vi "test Check for Invalid Section IDs.vi"(8 "error in (no error)":errorcluster, 11 "TestCase in":refnum<class "Routing and Faulting Scripting Unit Tests.lvclass">) -> (0 "error out":errorcluster, 3 "TestCase out":refnum<class "Routing and Faulting Scripting Unit Tests.lvclass">)   [LabVIEW 2017, in "Routing and Faulting Scripting Unit Tests.lvclass"]
uses:
  Routing and Faulting Scripting Unit Tests.lvclass
  <vilib>/NI Veristand/Custom Device API/Custom Device Item Ref.ctl
  Routing and Faulting Scripting Unit Tests.lvclass/Routing and Faulting Scripting Unit Tests.ctl
  Shared/Alias Mapping.ctl
  <vilib>/addons/_JKI Toolkits/VI Tester/TestCase.llb/TestCase.lvclass
  Routing and Faulting Scripting.lvlib
  Shared/Routing and Faulting Shared.lvlib
  <vilib>/NI VeriStand/Custom Device API/Custom Device API.lvlib
  C:/Program Files (x86)/National Instruments/LabVIEW 2017/vi.lib/addons/_JKI Toolkits/VI Tester/TestCase.llb/TestCase.lvclass
panel:
  in  "Save?":bool
  out "Output Filename":string
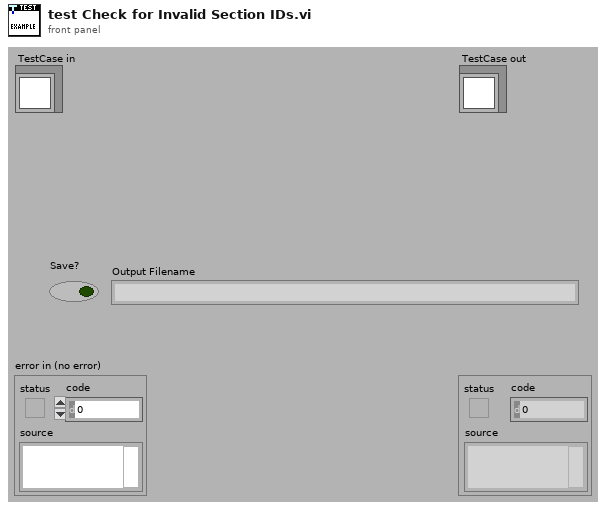
[diagram p1: front panel]
types:
  T1 = typedef "Custom Device API.lvlib/Custom Device Item Ref.ctl" = u64
  T2 = typedef "Routing and Faulting Shared.lvlib/Alias Mapping.ctl" = cluster{"Endpoint":string, "Alias":string}
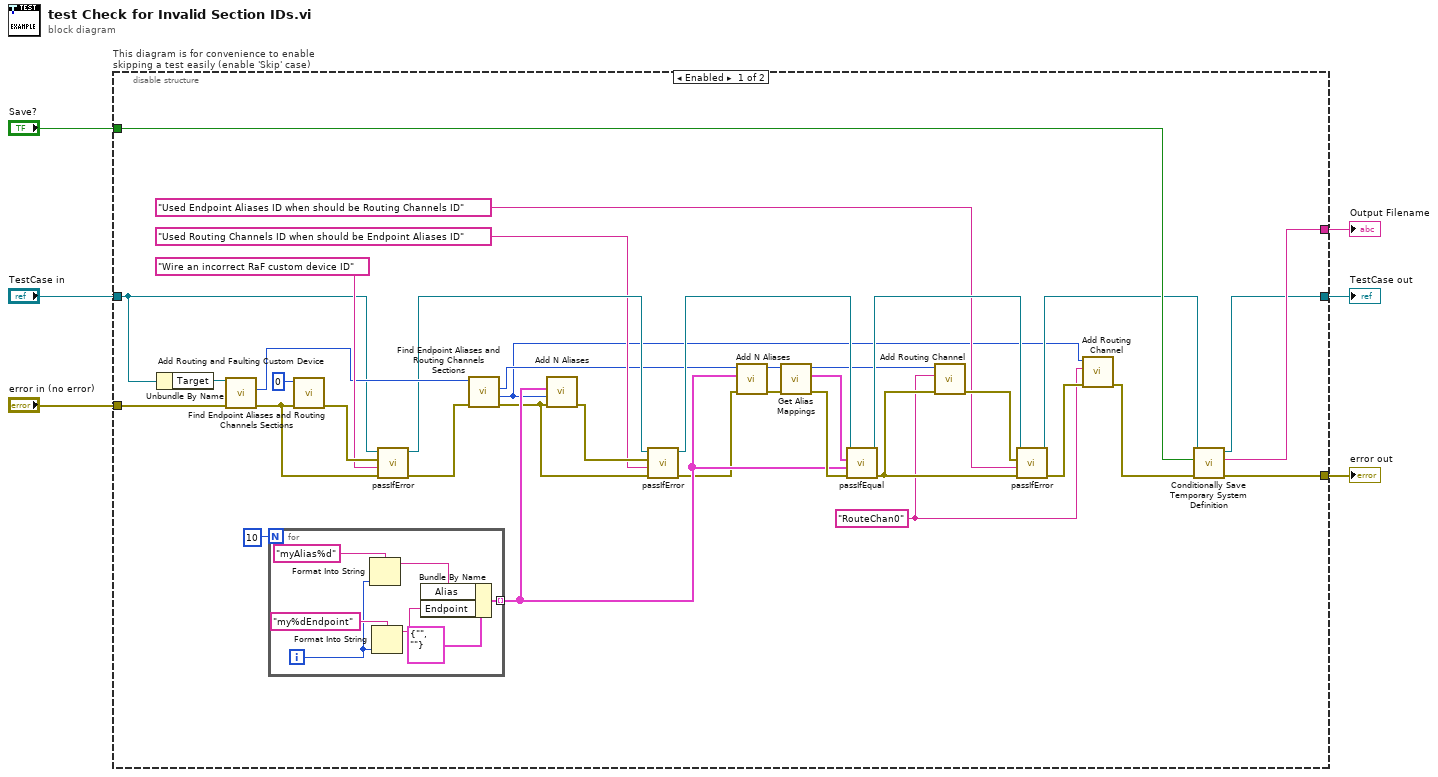
[diagram p0: block diagram]
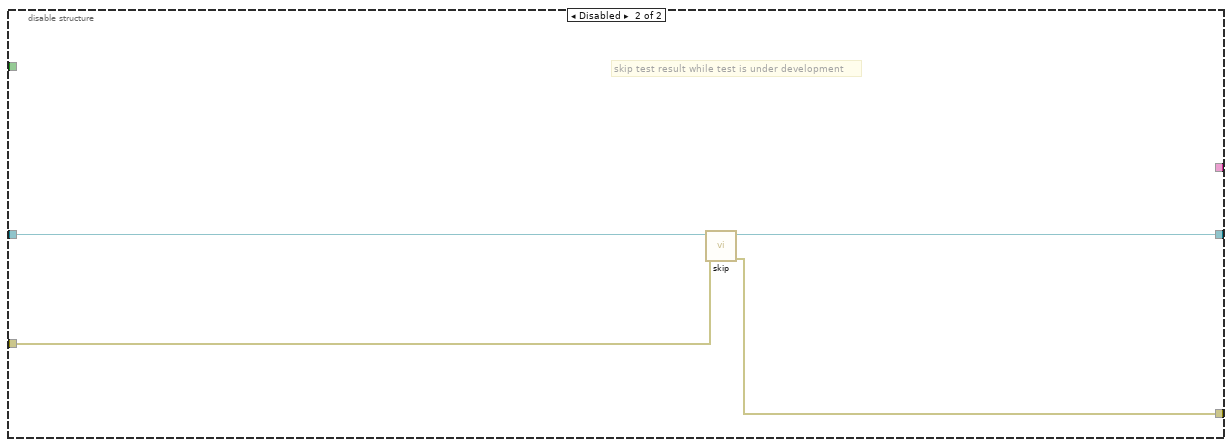
[diagram p2: hidden frame]
diagram:
  n1 = disable-structure "This diagram is for convenience to enable skipping a test easily (enable 'Skip' case)" shown="Enabled" {
    disable-tunnel: "TestCase in" -> [w25 w53]
    disable-tunnel: [w40 w51] -> w3
    disable-tunnel: [w41 w52] -> w5
    disable-tunnel: "error in (no error)" -> [w38 w50]
    disable-tunnel: [w42 _] -> w2
    disable-tunnel: "Save?" -> [w37 _]
    frame Enabled {
      w8 = "RouteChan0" ("Channel Name")
      n2 = Unbundle By Name(w25) -> ("Target"=w39:refnum<k24>)
      n3 = call "Add Routing and Faulting Custom Device.vi"("error in (no error)"=w38, "Target in"=w39) -> ("error out"=w31:errorcluster, "Routing and Faulting Custom Device Ref"=w28:T1)  [unwired: 7 in, 1 out]
      n4 = for {
        N: 10 -> [_]
        tunnel: [w43] -> w24 mode=indexing
        i -> [w47]
        n5 = Format Into String(format string="myAlias%d" ("Alias"), w47) -> (resulting string=w45:string)  [unwired: 2 in, 1 out]
        n6 = Format Into String(format string="my%dEndpoint" ("Alias"), w47) -> (resulting string=w44:string)  [unwired: 2 in, 1 out]
        n7 = Bundle By Name(cluster=T2 {"Endpoint"="", "Alias"=""} ("Alias Mapping"), "Alias"=w45, "Endpoint"=w44) -> (w43:T2)
      }
      n8 = call "Find Endpoint Aliases and Routing Channels Sections.vi"("error in (no error)"=w31, "Routing and Faulting Custom Device Ref in"=T1 0) -> ("error out"=w30:errorcluster)  [unwired: 6 in, 3 out]
      n9 = call-dynamic "passIfError.vi"("error in (no error)"=w31, "task (\"\")"="Wire an incorrect RaF custom device ID" ("task (\"\")"), "error"=w30, "TestCase in"=w25) -> ("error out"=w27:errorcluster, "TestCase out"=w23:refnum<class "Routing and Faulting Scripting Unit Tests.lvclass">)  [unwired: 6 in]
      n10 = call "Find Endpoint Aliases and Routing Channels Sections.vi"("error in (no error)"=w27, "Routing and Faulting Custom Device Ref in"=w28) -> ("error out"=w21:errorcluster, "Routing Channels Ref"=w7:T1, "Endpoint Aliases Ref"=w17:T1)  [unwired: 6 in, 1 out]
      n11 = call "Add N Aliases.vi"("error in (no error)"=w21, "Alias Mappings"=w24, "Endpoint Aliases Ref in"=w7) -> ("error out"=w20:errorcluster)  [unwired: 7 in, 1 out]
      n12 = call-dynamic "passIfError.vi"("error in (no error)"=w21, "task (\"\")"="Used Routing Channels ID when should be Endpoint Aliases ID" ("task (\"\")"), "error"=w20, "TestCase in"=w23) -> ("error out"=w18:errorcluster, "TestCase out"=w22:refnum<class "Routing and Faulting Scripting Unit Tests.lvclass">)  [unwired: 6 in]
      n13 = call "Add N Aliases.vi"("error in (no error)"=w18, "Alias Mappings"=w24, "Endpoint Aliases Ref in"=w17) -> ("error out"=w36:errorcluster, "Endpoint Aliases Ref out"=w35:T1)  [unwired: 7 in]
      n14 = call "Get Alias Mappings.vi"("error in (no error)"=w36, "Endpoint Aliases Ref in"=w35) -> ("error out"=w34:errorcluster, "Alias Mappings"=w33:T2[], "Endpoint Aliases Ref out"=w12:T1)  [unwired: 7 in]
      n15 = call-dynamic "passIfEqual.vi"("error in (no error)"=w34, "y"=w24, "x"=w33, "TestCase in"=w22) -> ("error out"=w14:errorcluster, "TestCase out"=w16:refnum<class "Routing and Faulting Scripting Unit Tests.lvclass">)  [unwired: 6 in]
      n16 = call "Add Routing Channel.vi"("error in (no error)"=w14, "Channel Name"=w8, "Routing Channels Ref in"=w12) -> ("error out"=w13:errorcluster)  [unwired: 6 in, 2 out]
      n17 = call-dynamic "passIfError.vi"("error in (no error)"=w14, "task (\"\")"="Used Endpoint Aliases ID when should be Routing Channels ID" ("task (\"\")"), "error"=w13, "TestCase in"=w16) -> ("error out"=w10:errorcluster, "TestCase out"=w15:refnum<class "Routing and Faulting Scripting Unit Tests.lvclass">)  [unwired: 6 in]
      n18 = call "Add Routing Channel.vi"("error in (no error)"=w10, "Channel Name"=w8, "Routing Channels Ref in"=w7) -> ("error out"=w9:errorcluster)  [unwired: 6 in, 2 out]
      n19 = call "Conditionally Save Temporary System Definition.vi"("error in (no error)"=w9, "Save?"=w37, "Test Case"=w15) -> ("error out"=w41:errorcluster, "filename"=w42:string, "Test Case"=w40:refnum<class "Routing and Faulting Scripting Unit Tests.lvclass">)  [unwired: 6 in]
    }
    frame Disabled {
      # "skip test result while test is under development"
      n20 = call <vilib>:"skip.vi"("error in (no error)"=w50, "TestCase in"=w53) -> ("error out"=w52:errorcluster, "TestCase out"=w51:refnum<class "Routing and Faulting Scripting Unit Tests.lvclass">)  [unwired: 8 in]
    }
  }
  "error out" <- w5
  "TestCase out" <- w3
  "Output Filename" <- w2
